vi "base64encode.vi"(4 "Error In":errorcluster, 7 "string in (not encoded)":string) -> (0 "Error Out":errorcluster, 3 "string out (base64-encoded)":string)   [LabVIEW 2015, in "Data Manipulation.lvlib"]
uses:
  Data Manipulation.lvlib
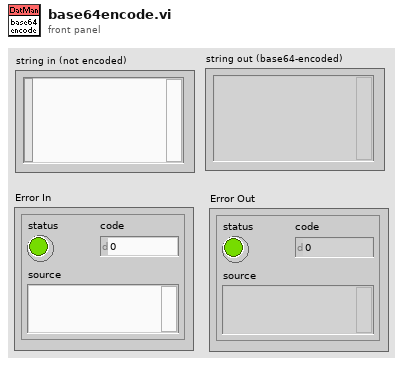
[diagram p1: front panel]
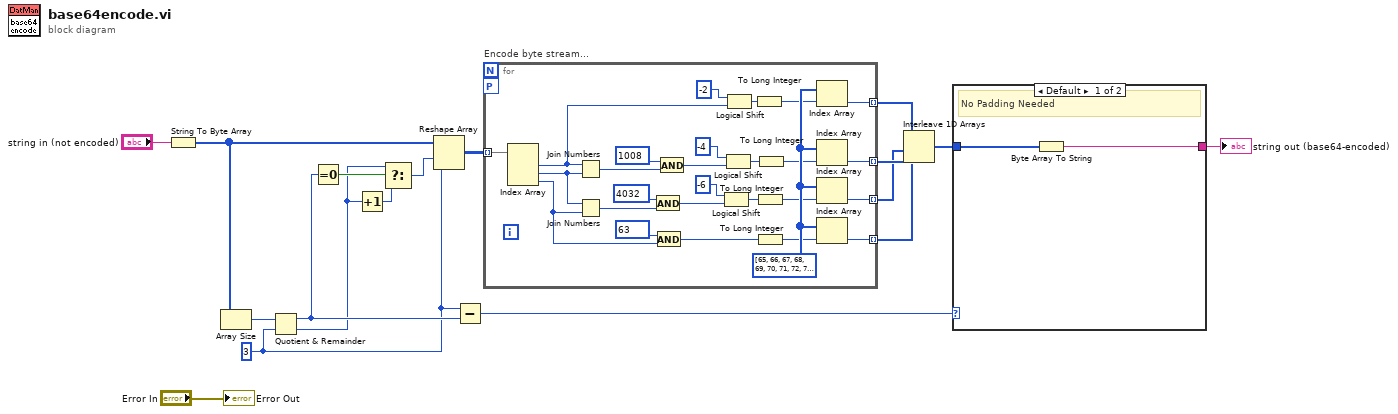
[diagram p0: block diagram]
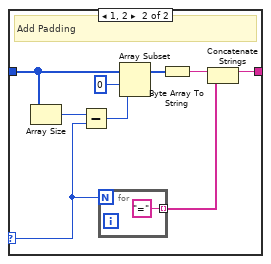
[diagram p2: hidden frame]
diagram:
  w1 = 3 ("y")
  n1 = String To Byte Array(string="string in (not encoded)") -> (unsigned byte array=w5:u8[])
  n2 = Array Size(array=w5) -> (size(s)=w13:i32)
  n3 = Quotient & Remainder(x=w13, y=w1) -> (x-y*floor(x/y)=w14:i32, floor(x/y)=w7:i32)
  n4 = Equal To 0?(x=w14) -> (x = 0?=w15:bool)
  n5 = Increment(x=w7) -> (x+1=w8:i32)
  n6 = Select(t=w7, s=w15, f=w8) -> (s? t:f=w4:i32)
  n7 = Reshape Array(w5, w4, w1) -> (w3:u8[][])
  n8 = Subtract(x=w1, y=w14) -> (x-y=w2:i32)
  n9 = for "Encode byte stream..." {
    tunnel: [w28] -> w9 mode=indexing
    tunnel: [w29] -> w10 mode=indexing
    tunnel: [w30] -> w11 mode=indexing
    tunnel: [w31] -> w12 mode=indexing
    workers-P: _ -> [_]
    tunnel: w3 -> [w22] mode=indexing
    w27 = u8[] [65, 66, 67, 68, 69, 70, 71, 72, 73, 74, 75, 76, 77, 78, 79, 80, 81, 82, 83, 84, 85, 86, 87, 88, 89, 90, 97, 98, 99, 100, 101, 102, 103, 104, 105, 106, 107, 108, 109, 110, 111, 112, 113, 114, 115, 116, 117, 118, 119, 120, 121, 122, 48, 49, 50, 51, 52, 53, 54, 55, 56, 57, 43, 47] ("unsigned byte array")
    n10 = Index Array(array=w22) -> (element #1=w21:u8, element #2=w20:u8, element #3=w19:u8)  [unwired: 3 in]
    n11 = Join Numbers(hi=w21, lo=w20) -> ((hi.lo)=w44:u16)
    n12 = Join Numbers(hi=w20, lo=w19) -> ((hi.lo)=w40:u16)
    n13 = And(x=u16 4032, y=w40) -> (x .and. y?=w38:u16)
    n14 = And(x=u8 63, y=w19) -> (x .and. y?=w32:u8)
    n15 = And(x=u16 1008, y=w44) -> (x .and. y?=w42:u16)
    n16 = Logical Shift(y=i8 -6, x=w38) -> (x << y=w33:u16)
    n17 = Logical Shift(y=i8 -4, x=w42) -> (x << y=w34:u16)
    n18 = Logical Shift(y=i8 -2, x=w21) -> (x << y=w35:u8)
    n19 = To Long Integer(number=w35) -> (32bit integer=w23:i32)
    n20 = To Long Integer(number=w33) -> (32bit integer=w25:i32)
    n21 = To Long Integer(number=w32) -> (32bit integer=w26:i32)
    n22 = To Long Integer(number=w34) -> (32bit integer=w24:i32)
    n23 = Index Array(array=w27, index=w23) -> (element=w31:u8)
    n24 = Index Array(array=w27, index=w24) -> (element=w30:u8)
    n25 = Index Array(array=w27, index=w25) -> (element=w29:u8)
    n26 = Index Array(array=w27, index=w26) -> (element=w28:u8)
  }
  n27 = Interleave 1D Arrays(w12, w11, w10, w9) -> (w6:u8[])
  n28 = case shown="Default" w2 {
    selector: w2 -> [_ w52]
    tunnel: [w46 w49] -> w16
    tunnel: w6 -> [w47 w53]
    frame Default {
      # "No Padding Needed"
      n29 = Byte Array To String(unsigned byte array=w47) -> (string=w46:string)
    }
    frame 1, 2 {
      # "Add Padding"
      n30 = Array Size(array=w53) -> (size(s)=w54:i32)
      n31 = Subtract(x=w54, y=w52) -> (x-y=w50:i32)
      n32 = for {
        N: w52 -> [_]
        tunnel: ["="] -> w48 mode=indexing
      }
      n33 = Array Subset(array=w53, index=0, length=w50) -> (w56:u8[])
      n34 = Byte Array To String(unsigned byte array=w56) -> (string=w55:string)
      n35 = Concatenate Strings(w55, w48) -> (w49:string)
    }
  }
  "string out (base64-encoded)" <- w16
  "Error Out" <- "Error In"
